vi "SQLite Query - Insert.vi"(8 "error in":errorcluster, 9 "Data":string[](array[string]), 10 "Table Headers":string[](array[string]), 11 "Table Name":string) -> (0 "error out":errorcluster, 3 "SQLite Query":string)   [LabVIEW 2014, in "TableLogger_SQLite_Actor.lvlib" / "TableLogger_SQLite_Actor.lvclass"]
uses:
  TableLogger_SQLite_Actor.lvclass
panel:
  # "Connector Pane"
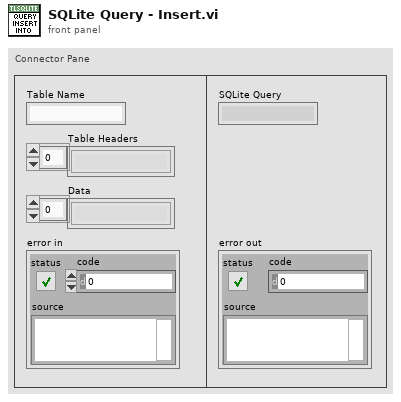
[diagram p1: front panel]
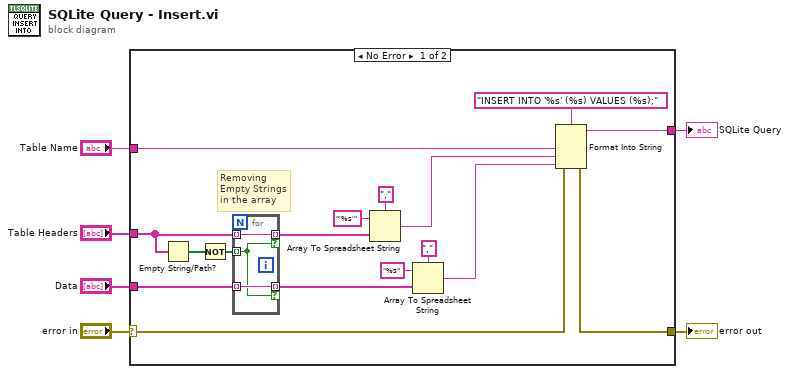
[diagram p0: block diagram]
diagram:
  n1 = case shown="No Error" "error in" {
    selector: "error in" -> [w16 w27]
    tunnel: "Data" -> [w10 _]
    tunnel: [w23 _] -> w5
    tunnel: "Table Name" -> [w18 _]
    tunnel: "Table Headers" -> [w12 _]
    tunnel: [w15 w27] -> w1
    frame No Error {
      # "Removing Empty Strings in the array"
      n2 = Empty String/Path?(string/path=w12) -> (empty?=w20:bool[])
      n3 = Not(x=w20) -> (.not. x?=w21:bool[])
      n4 = for {
        tunnel: w21 -> [w24] mode=indexing
        tunnel: w12 -> [w26] mode=indexing
        tunnel: [w26] -> w8 mode=indexing if=w24
        tunnel: [w25] -> w9 mode=indexing if=w24
        tunnel: w10 -> [w25] mode=indexing
      }
      n5 = Array To Spreadsheet String(delimiter (Tab)=",", array=w8, 3:"'%s'" ("format string")) -> (spreadsheet string=w11:string)
      n6 = Array To Spreadsheet String(delimiter (Tab)=",", array=w9, 3:"%s" ("format string")) -> (spreadsheet string=w7:string)
      n7 = Format Into String(format string="INSERT INTO '%s' (%s) VALUES (%s);" ("SQL"), error in=w16, w18, w11, w7) -> (resulting string=w23:string, error out=w15:errorcluster)  [unwired: 1 in]
    }
    frame Error {
    }
  }
  "SQLite Query" <- w5
  "error out" <- w1
